vi "Glue Fiducials.vi"() -> ()   [LabVIEW 2020]
uses:
  Controller/Dispenser/Dispenser.lvclass
  Controller/Controller.lvclass
  Aerotech.lvlib
  Dispense.lvclass
panel:
  in  "Z speed":dbl
  in  "Z1":dbl
  in  "z up":dbl
  in  "XY End point":dbl[](array[numeric])
  in  "XY Starting Point":dbl[](array[numeric])
  in  "XY speed":dbl
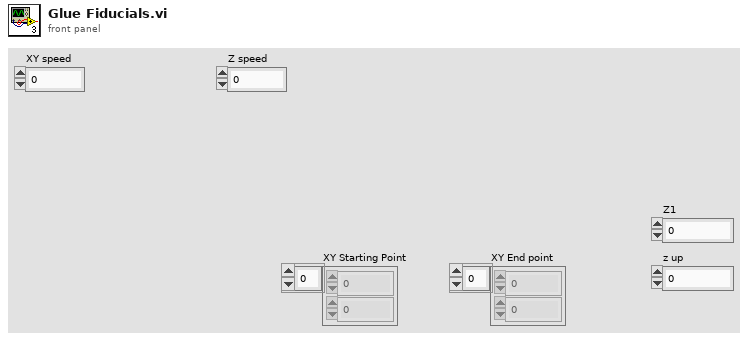
[diagram p1: front panel]
types:
  T1 = typedef "Controller.lvclass/Controllers.ctl" = cluster{"I-O.lvclass":refnum<class "I-O.lvclass">, "Dispenser.lvclass":refnum<class "Dispenser.lvclass">, "Gantry":refnum<k24>}
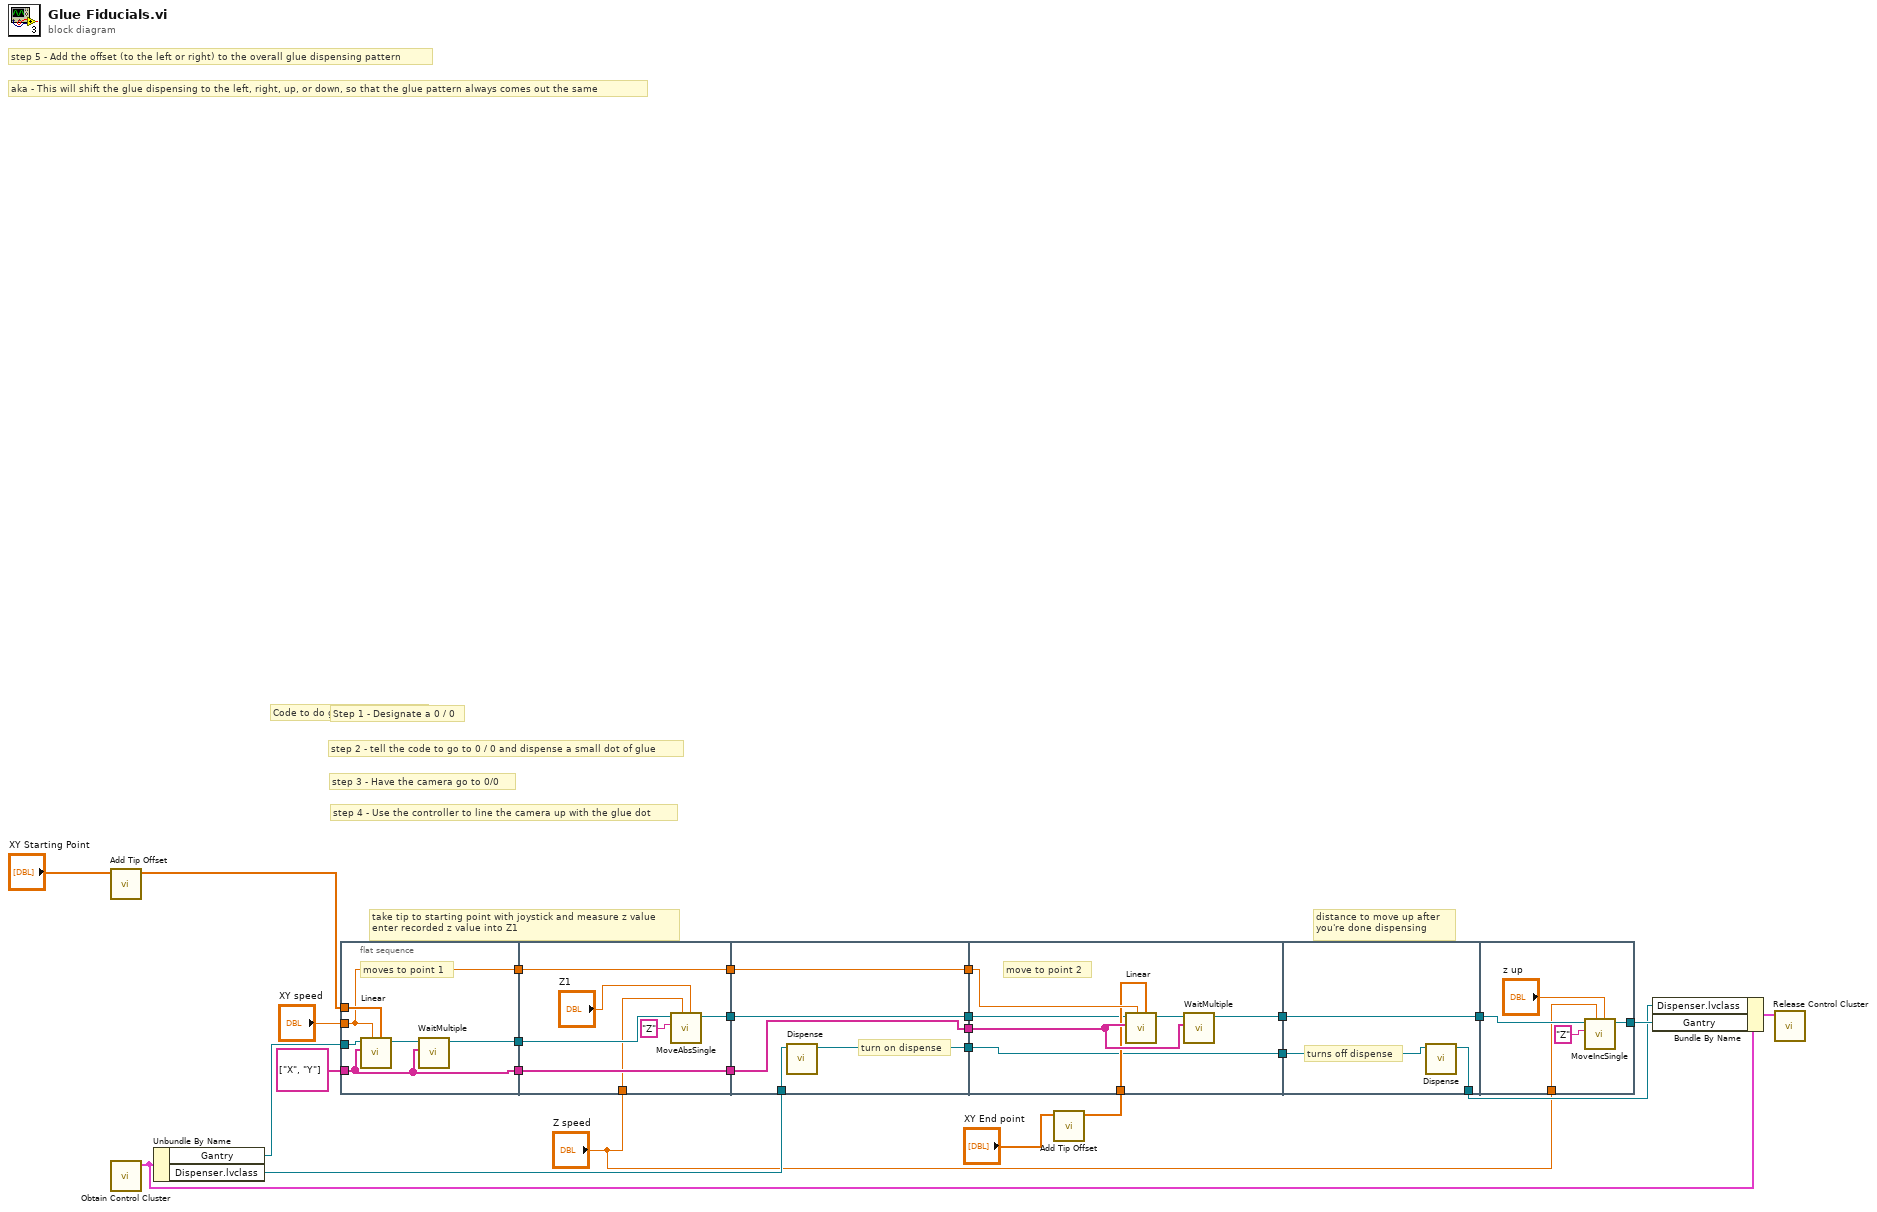
[diagram p0: block diagram]
diagram:
  # "distance to move up after \nyou're done dispensing"
  # "take tip to starting point with joystick and measure z value\nenter recorded z value into Z1"
  # "aka - This will shift the glue dispensing to the left, right, up, or down, so that the glue pattern always comes out the same"
  # "step 5 - Add the offset (to the left or right) to the overall glue dispensing pattern"
  # "step 4 - Use the controller to line the camera up with the glue dot"
  # "step 3 - Have the camera go to 0/0"
  # "step 2 - tell the code to go to 0 / 0 and dispense a small dot of glue"
  # "Step 1 - Designate a 0 / 0"
  # "Code to do glue test fiducials"
  n1 = call "Add Tip Offset.vi"("XYZTheta"="XY Starting Point") -> ("XYZTheta"=w22:dbl[])  [unwired: 10 in]
  n2 = call "Obtain Control Cluster.vi"() -> ("Control Out"=w12:T1)  [unwired: 11 in]
  n3 = Unbundle By Name(w12) -> ("Gantry"=w26:refnum<k24>, "Dispenser.lvclass"=w21:refnum<class "Dispenser.lvclass">)
  n4 = flat-sequence {
    tunnel: w26 -> [w32]
    tunnel: "XY speed" -> [w27]
    tunnel: string[] ["X", "Y"] ("axis names") -> [w28]
    tunnel: w22 -> [w30]
    tunnel: [w29] -> w8
    tunnel: [w28] -> w7
    tunnel: [w27] -> w5
    tunnel: w8 -> [w36]
    tunnel: w7 -> [w39]
    tunnel: [w39] -> w6
    tunnel: w5 -> [w38]
    tunnel: [w38] -> w4
    tunnel: [w35] -> w3
    tunnel: "Z speed" -> [w33]
    tunnel: w21 -> [w44]
    tunnel: w6 -> [w43]
    tunnel: [w43] -> w20
    tunnel: w4 -> [w42]
    tunnel: [w42] -> w19
    tunnel: [w41] -> w16
    tunnel: w3 -> [w40]
    tunnel: [w40] -> w2
    tunnel: w20 -> [w50]
    tunnel: w19 -> [w49]
    tunnel: w17 -> [w48]
    tunnel: w16 -> [w47]
    tunnel: [w47] -> w15
    tunnel: [w46] -> w14
    tunnel: w2 -> [w45]
    tunnel: w15 -> [w54]
    tunnel: w14 -> [w53]
    tunnel: [w53] -> w13
    tunnel: [w52] -> w10
    tunnel: w13 -> [w58]
    tunnel: [w57] -> w11
    tunnel: "Z speed" -> [w55]
    frame #0 {
      # "moves to point 1"
      n5 = call "Linear.vi"("distances"=w30, "speed"=w27, "axis names"=w28, "controller in"=w32) -> ("controller out"=w31:refnum<k24>)  [unwired: 6 in, 1 out]
      n6 = call "WaitMultiple.vi"("axis names"=w28, "controller in"=w31) -> ("controller out"=w29:refnum<k24>)  [unwired: 7 in, 2 out]
    }
    frame #1 {
      n7 = call "MoveAbsSingle.vi"("position"="Z1", "speed"=w33, "axis name"="Z", "controller in"=w36) -> ("controller out"=w35:refnum<k24>)  [unwired: 6 in, 1 out]
    }
    frame #2 {
      # "turn on dispense"
      n8 = call-dynamic "Dispense.vi"("Dispenser in"=w44) -> ("Dispenser out"=w41:refnum<class "Dispenser.lvclass">)  [unwired: 9 in, 1 out]
    }
    frame #3 {
      # "move to point 2"
      n9 = call "Linear.vi"("distances"=w48, "speed"=w49, "axis names"=w50, "controller in"=w45) -> ("controller out"=w51:refnum<k24>)  [unwired: 6 in, 1 out]
      n10 = call "WaitMultiple.vi"("axis names"=w50, "controller in"=w51) -> ("controller out"=w46:refnum<k24>)  [unwired: 7 in, 2 out]
    }
    frame #4 {
      # "turns off dispense"
      n11 = call-dynamic "Dispense.vi"("Dispenser in"=w54) -> ("Dispenser out"=w52:refnum<class "Dispenser.lvclass">)  [unwired: 9 in, 1 out]
    }
    frame #5 {
      n12 = call "MoveIncSingle.vi"("distance"="z up", "speed"=w55, "axis name"="Z", "controller in"=w58) -> ("controller out"=w57:refnum<k24>)  [unwired: 6 in, 1 out]
    }
  }
  n13 = call "Add Tip Offset.vi"("XYZTheta"="XY End point") -> ("XYZTheta"=w17:dbl[])  [unwired: 10 in]
  n14 = Bundle By Name(cluster=w12, "Dispenser.lvclass"=w10, "Gantry"=w11) -> (w9:T1)
  n15 = call "Release Control Cluster.vi"("output cluster"=w9) -> ()  [unwired: 11 in]
